vi "HelloWord Client.vi"() -> ()   [LabVIEW 2014]
uses:
  <vilib>/addons/zeromq/socket_type.ctl
  <vilib>/addons/zeromq/zmq_context.lvclass
  <vilib>/addons/zeromq/zeromq.lvlib
  <vilib>/addons/zeromq/zmq_socket.lvclass
panel:
  out "data from sever":string
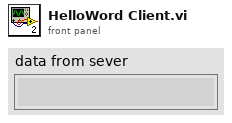
[diagram p1: front panel]
types:
  T1 = typedef "zeromq.lvlib/socket_type.ctl" = enum8{"ZMQ_PAIR", "ZMQ_PUB", "ZMQ_SUB", "ZMQ_REQ", "ZMQ_REP", "ZMQ_DEALER", "ZMQ_ROUTER", "ZMQ_PULL", "ZMQ_PUSH", "ZMQ_XPUB", "ZMQ_XSUB"}
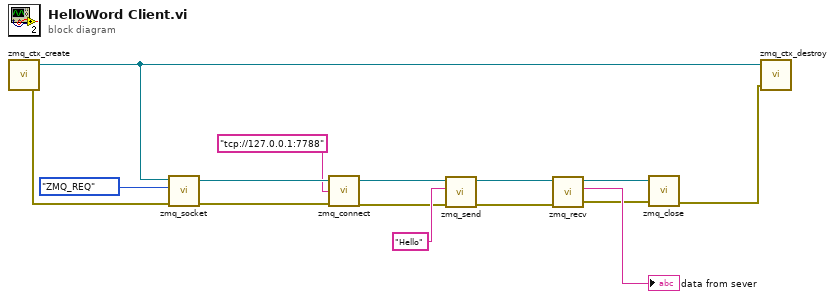
[diagram p0: block diagram]
diagram:
  n1 = call <vilib>:"zmq_ctx_create.vi"() -> ("error out"=w14:errorcluster, "context out"=w13:refnum<class "zmq_context.lvclass">)  [unwired: 4 in]
  n2 = call <vilib>:"zmq_socket.vi"("error in"=w14, "socket type"=socket_type."ZMQ_REQ", "context in"=w13) -> ("error out"=w11:errorcluster, "socket out"=w12:refnum<class "zmq_socket.lvclass">)  [unwired: 2 in, 1 out]
  n3 = call <vilib>:"zmq_connect.vi"("error in"=w11, "endpoint"="tcp://127.0.0.1:7788", "socket in"=w12) -> ("error out"=w5:errorcluster, "socket out"=w6:refnum<class "zmq_socket.lvclass">)  [unwired: 1 in]
  n4 = call <vilib>:"zmq_send.vi"("error in"=w5, "data"="Hello", "socket in"=w6) -> ("error out"=w4:errorcluster, "socket out"=w3:refnum<class "zmq_socket.lvclass">)  [unwired: 4 in]
  n5 = call <vilib>:"zmq_recv.vi"("error in"=w4, "socket in"=w3) -> ("error out"=w1:errorcluster, "data"=→"data from sever":string, "socket out"=w2:refnum<class "zmq_socket.lvclass">)  [unwired: 3 in, 2 out]
  n6 = call <vilib>:"zmq_close.vi"("error in"=w1, "socket"=w2) -> ("error out"=w7:errorcluster)  [unwired: 3 in]
  n7 = call <vilib>:"zmq_ctx_destroy.vi"("error in"=w7, "context in"=w13) -> ()  [unwired: 3 in, 1 out]
